vi "Read Data Type.vi"(8 "error in (no error)":errorcluster, 11 "OnChange_Boolean in":refnum<class "OnChange_Boolean.lvclass">) -> (0 "error out":errorcluster, 2 "Abs_Boolean.lvclass":refnum<class "Abs_Boolean.lvclass">, 3 "OnChange_Boolean out":refnum<class "OnChange_Boolean.lvclass">)   [LabVIEW 2021, in "OnChange_Boolean.lvclass"]
uses:
  OnChange_Boolean.lvclass
  <vilib>/TSA/Abstract Data Classes/Abs_Types/Boolean/Abs_Boolean.lvclass
  OnChange_Boolean.lvclass/OnChange_Boolean.ctl
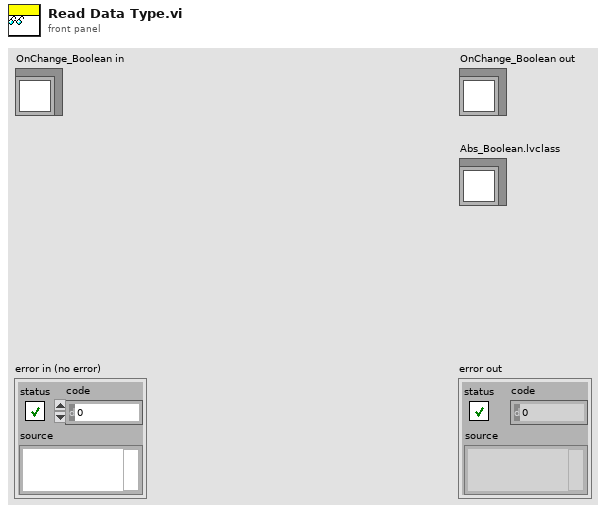
[diagram p1: front panel]
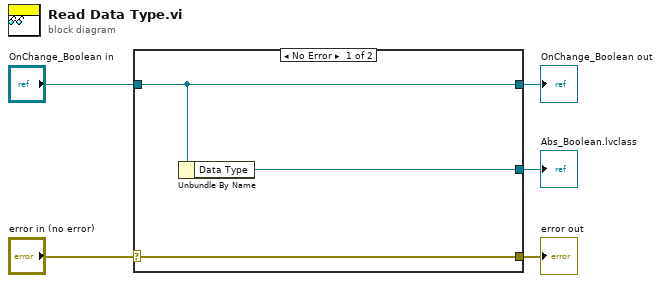
[diagram p0: block diagram]
diagram:
  n1 = case shown="No Error" "error in (no error)" {
    selector: "error in (no error)" -> [w8 w9]
    tunnel: [w8 w9] -> w4
    tunnel: [w7 w10] -> w2
    tunnel: "OnChange_Boolean in" -> [w7 w10]
    tunnel: [w6 _] -> w1
    frame No Error {
      n2 = Unbundle By Name(w7) -> ("Data Type"=w6:refnum<class "Abs_Boolean.lvclass">)
    }
    frame Error {
    }
  }
  "error out" <- w4
  "OnChange_Boolean out" <- w2
  "Abs_Boolean.lvclass" <- w1
